vi "Receive Q.vi"(8 "error in (no error)":errorcluster, 10 "Disp Data":dbl[](array[numeric]), 11 "Task Viewer in":refnum<class "Task Viewer.lvclass">) -> (0 "error out":errorcluster, 3 "Task Viewer out":refnum<class "Task Viewer.lvclass">)   [LabVIEW 2020, in "Task Viewer.lvlib" / "Task Viewer.lvclass"]
uses:
  Task Viewer.lvclass
  Task Viewer.lvclass/Task Viewer.ctl
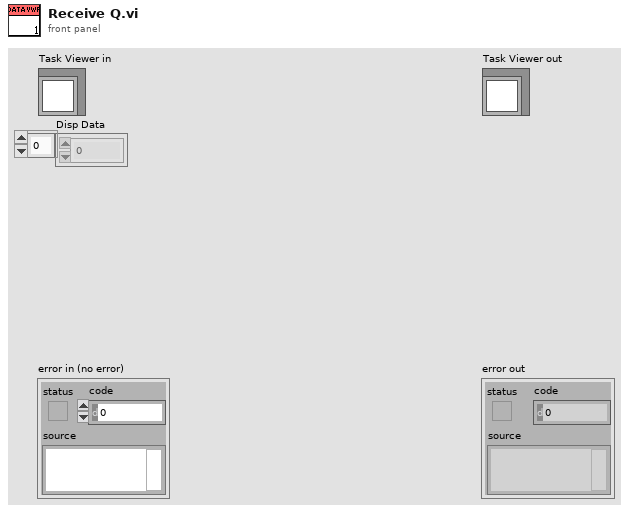
[diagram p1: front panel]
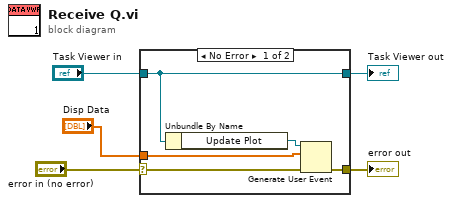
[diagram p0: block diagram]
diagram:
  n1 = case shown="No Error" "error in (no error)" {
    selector: "error in (no error)" -> [w8 w12]
    tunnel: [w9 w12] -> w4
    tunnel: [w7 w11] -> w2
    tunnel: "Task Viewer in" -> [w7 w11]
    tunnel: "Disp Data" -> [w6 _]
    frame No Error {
      n2 = Unbundle By Name(w7) -> ("Update Plot"=w10:refnum<user-event>)
      n3 = Generate User Event(user event=w10, event data cluster=w6, error in=w8) -> (error out=w9:errorcluster)  [unwired: 1 in, 1 out]
    }
    frame Error {
    }
  }
  "error out" <- w4
  "Task Viewer out" <- w2
